vi "Import Pictures from Folder.vi"(0 "Display State In":T1, 5 "Maximum":i32=100, 7 "Pictures Folder":path, 9 "Container State":T3, 11 "error in (no error)":errorcluster) -> (4 "Display State Out":T1, 15 "error out":errorcluster)   [LabVIEW 2016]
uses:
  <vilib>/Utility/miscctls.llb/LVBoundsTypeDef.ctl
  HorizontalList.xctl
  <vilib>/_xctls/Container State.ctl
  <vilib>/_xctls/XControlSupport.lvlib
  HorizontalList_State.ctl
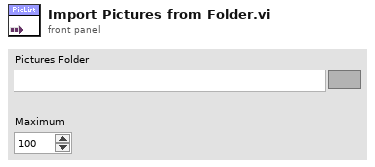
[diagram p1: front panel]
types:
  T1 = typedef "HorizontalList.xctl/HorizontalList_State.ctl" = cluster{"Persistent":cluster{"Elements":string[], "PicElements":picture[], "Limits":i32[], "Selection":picture[], "Selection Color":u32, "Highlight":picture[], "Highlight Val":i32, "Highlight Color":u32}, "Draw Area Size":T2, "List Ref":refnum<vi>, "Visible":u8}
  T2 = typedef "LVBoundsTypeDef.ctl" = cluster{"Width":u32, "Height":u32}
  T3 = typedef "XControlSupport.lvlib/Container State.ctl" = cluster{"Indicator?":bool, "Run Mode?":bool, " Refnum":refnum<vi>}
  T4 = typedef "imagedata.ctl" = cluster{"image type":i32, "image depth":i32, "image":u8[], "mask":u8[], "colors":u32[], "Rectangle":cluster{"left":i16, "top":i16, "right":i16, "bottom":i16}}
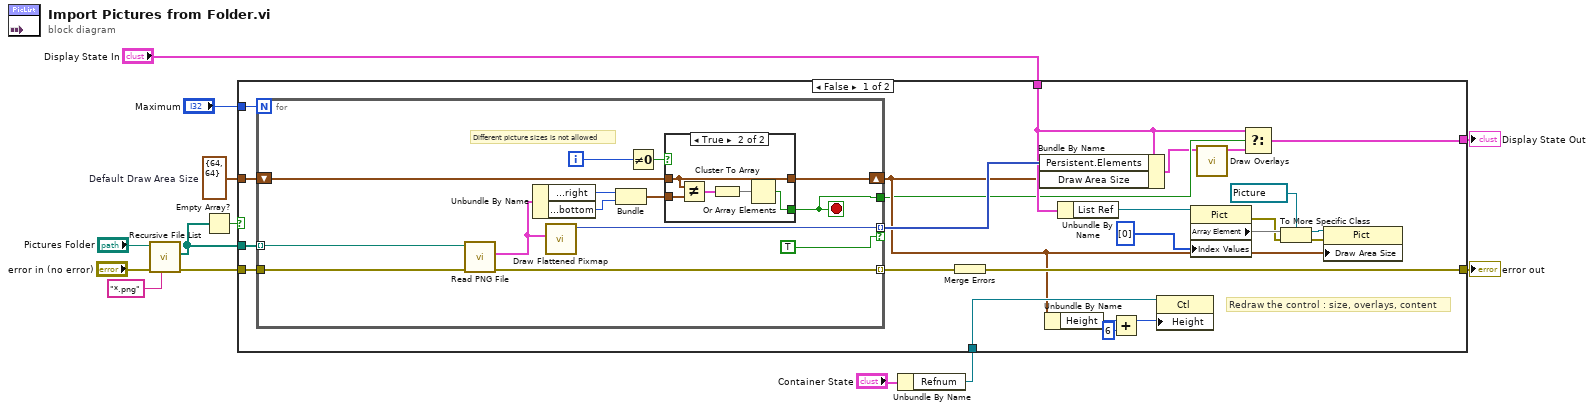
[diagram p0: block diagram]
diagram:
  w7 = T2 {"Width"=64, "Height"=64}  # Default Draw Area Size
  n1 = call <vilib>:"Recursive File List.vi"("pattern"="*.png", "error in (no error)"="error in (no error)", "Folder Path"="Pictures Folder") -> ("error out"=w5:errorcluster, "All Files in Dir"=w4:path[])  [unwired: 4 in, 3 out]
  n2 = Empty Array?(array=w4) -> (empty?=w10:bool)
  n3 = Unbundle By Name("Container State") -> ("Refnum"=w2:refnum<vi>)
  n4 = case shown="False" w10 {
    tunnel: w4 -> [w37 _]
    tunnel: w5 -> [w36 w59]
    tunnel: [w33 w59] -> w8
    tunnel: w7 -> [w32 _]
    tunnel: [w31 w58] -> w9
    tunnel: "Display State In" -> [w30 w58]
    tunnel: w2 -> [w24 _]
    tunnel: "Maximum" -> [w14 _]
    frame False {
      # "Redraw the control : size, overlays, content"
      n5 = for {
        N: w14 -> [_]
        tunnel: w37 -> [w51] mode=indexing
        tunnel: w36 -> [w50]
        tunnel: [w49] -> w35 mode=indexing if=TRUE
        tunnel: [w48] -> w34 mode=indexing
        shift-right: [w45] -> w23
        shift-left: w32 -> [w46]
        tunnel: [w44] -> w22
        i -> [w47]
        stop <- w44 stop-if-true
        # "Different picture sizes is not allowed"
        n6 = call <vilib>:"Read PNG File.vi"("error in (no error)"=w50, "path to PNG file"=w51) -> ("error out"=w48:errorcluster, "image data"=w42:T4)  [unwired: 7 in, 1 out]
        n7 = Unbundle By Name(w42) -> ("Rectangle.right"=w41:i16, "Rectangle.bottom"=w40:i16)
        n8 = call <vilib>:"Draw Flattened Pixmap.vi"("image data"=w42) -> ("new picture"=w49:picture)  [unwired: 8 in]
        n9 = Bundle("right"=w41, "bottom"=w40) -> (w38:cluster{"right":i16, "bottom":i16})  [unwired: 1 in]
        n10 = Not Equal To 0?(x=w47) -> (x != 0?=w39:bool)
        n11 = case shown="True" w39 {
          tunnel: w46 -> [_ w57]
          tunnel: [w52 w57] -> w45
          tunnel: w38 -> [w52 w56]
          tunnel: [_ w53] -> w44
          frame False {
          }
          frame True {
            n12 = Not Equal?(x=w57, y=w56) -> (x != y?=w55:cluster{bool, bool})
            n13 = Cluster To Array(cluster=w55) -> (array=w54:bool[])
            n14 = Or Array Elements(Boolean array=w54) -> (logical OR=w53:bool)
          }
        }
      }
      n15 = Merge Errors(w34) -> (w33:errorcluster)
      n16 = Bundle By Name(cluster=w30, "Persistent.Elements"=w35, "Draw Area Size"=w23) -> (w17:T1)
      n17 = Unbundle By Name(w23) -> ("Height"=w21:u32)
      n18 = Unbundle By Name(w30) -> ("List Ref"=w29:refnum<vi>)
      n19 = Add(x=w21, y=u32 6) -> (x+y=w20:u32)
      n20 = property class="Ctl"(reference=w24, "Height"=w20) -> ()  [unwired: 1 in, 2 out]
      n21 = property class="Pict"(reference=w29, "Index Values"=u32[] [0]) -> (error out=w15:errorcluster, "Array Element"=w28)  [unwired: 1 in, 1 out]
      n22 = call "Draw Overlays.vi"("Default Control State in"=w17) -> ("Default Control State out"=w16:T1)  [unwired: 10 in]
      n23 = Select(t=w30, s=w22, f=w16) -> (s? t:f=w31:T1)
      n24 = To More Specific Class(target class=refnum<vi> refnum ("reference"), reference=w28, error in=w15) -> (specific class reference=w26:refnum<vi>, error out=w25:errorcluster)
      n25 = property class="Pict"(reference=w26, error in=w25, "Draw Area Size"=w23) -> ()  [unwired: 2 out]
    }
    frame True {
    }
  }
  "Display State Out" <- w9
  "error out" <- w8
